vi "Offset Rectangle.vi"() -> ()   [LabVIEW 2012]
uses:
  demo dll.dll
panel:
  out "Offset Rect":T1
  in  "dy":i32
  in  "dx":i32
  in  "Rect":T1
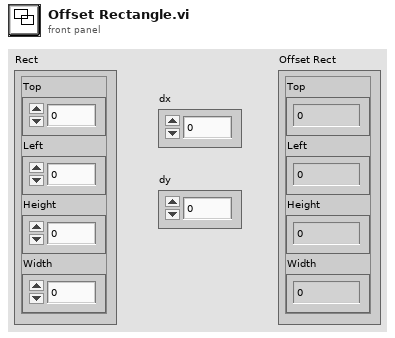
[diagram p1: front panel]
types:
  T1 = cluster{"Top":i32, "Left":i32, "Height":i32, "Width":i32}
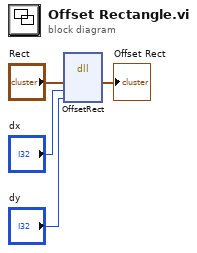
[diagram p0: block diagram]
diagram:
  n1 = dll-call lib="PTH1+abs EBOOK\t功能块DLLdemo dll.dll" fn="OffsetRect"("Rect"="Rect", "dx"="dx", "dy"="dy") -> ("Rect"=→"Offset Rect":T1)  [unwired: 6 in, 2 out]
